vi "Untitled 1.vi"(2 "rate":dbl=2.0, 3 "number of samples":i32=10, 4 "timeout (s)":dbl=10.0 format="%0.2f", 5 "error in":errorcluster, 7 "stop (T)":bool=TRUE) -> (14 "task out":refnum<k21>, 15 "data":dynamicdata(graph), 19 "error out":errorcluster)   [LabVIEW 2024]
doc: "Creates, edits, and runs tasks using NI-DAQmx. Refer to the NI-DAQmx Readme for a complete listing of devices NI-DAQmx supports.\n\nWhen you place this Express VI on the block diagram, the DAQ Assistant launches to create a new task. After you create a task, you can double-click the DAQ Assistant Express VI to edit that task. For continuous measurement or generation, place a while loop around the DAQ Assistant Express VI."
uses:
  <vilib>/DAQmx/read.llb/DAQmx Read.vi
  <vilib>/DAQmx/read.llb/DAQmx Read (Analog 1D Wfm NChan NSamp).vi
  <vilib>/DAQmx/create/channels.llb/DAQmx Create Channel (TEDS-AI-Current-Basic).vi
  <vilib>/DAQmx/create/channels.llb/DAQmx Create Channel (AI-Current-Basic).vi
  <vilib>/DAQmx/create/channels.llb/DAQmx Create Channel (TEDS-AI-Voltage-Basic).vi
  <vilib>/DAQmx/create/channels.llb/DAQmx Create Channel (AI-Voltage-Basic).vi
  <vilib>/DAQmx/configure/timing.llb/DAQmx Timing (Sample Clock).vi
  <vilib>/DAQmx/miscellaneous.llb/DAQmx Fill In Error Info.vi
  <resource>/objmgr/daqmx.rc
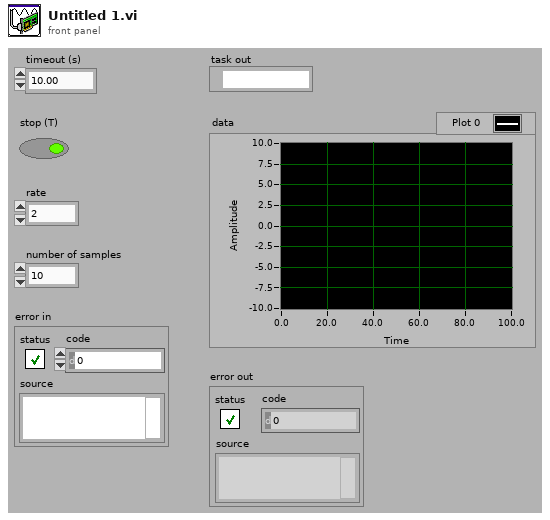
[diagram p1: front panel]
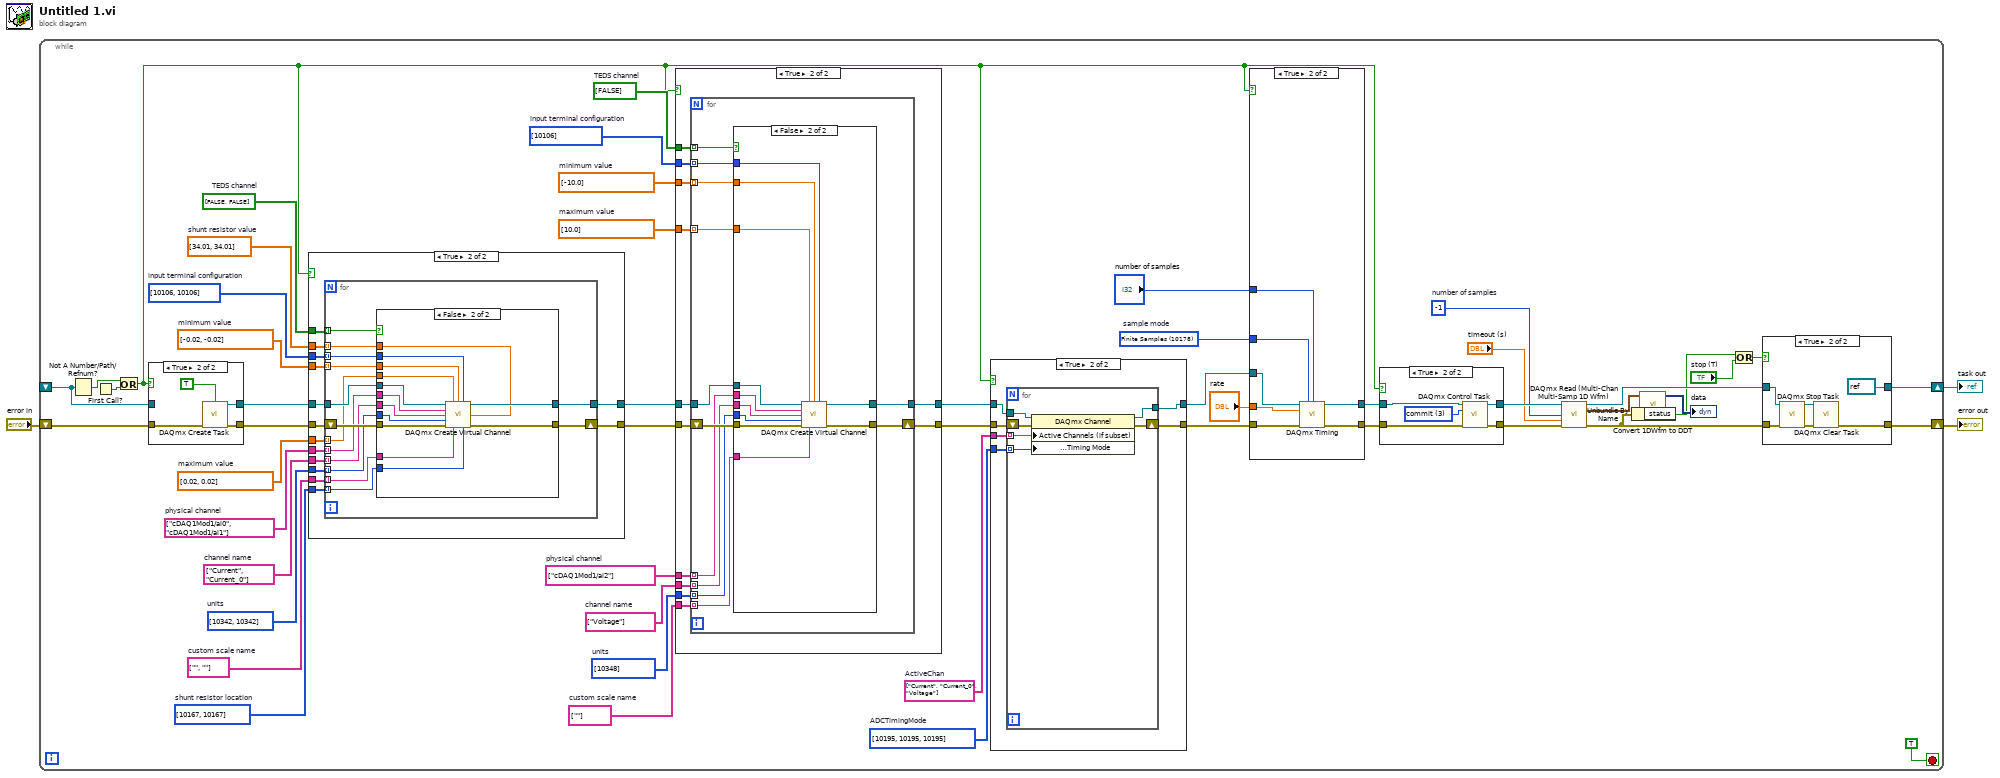
[diagram p0: block diagram]
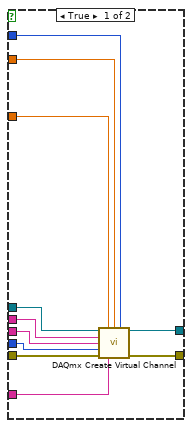
[diagram p7: hidden frame]
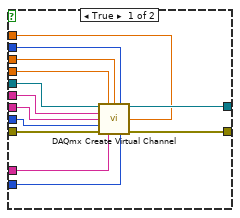
[diagram p9: hidden frame]
diagram:
  n1 = while {
    shift-right: [w10] -> w1
    shift-left: _ -> [w52]
    shift-right: [w8] -> w2
    shift-left: "error in" -> [w53]
    stop <- TRUE stop-if-true
    w14 = -1  # number of samples
    w20 = 10178 items=["Finite Samples"=10178, "Continuous Samples"=10123, "Hardware Timed Single Point"=12522]  # sample mode
    w26 = i32[] [10195, 10195, 10195] items=["High Resolution"=10195, "High Speed"=14712, "Best 50 Hz Rejection"=14713, "Best 60 Hz Rejection"=14714]  # ADCTimingMode
    w27 = string[] ["Current", "Current_0", "Voltage"]  # ActiveChan
    w29 = bool[] [FALSE]  # TEDS channel
    w30 = string[] [""]  # custom scale name
    w31 = i32[] [10348] items=["Volts"=10348, "From TEDS"=12516, "From Custom Scale"=10065]  # units
    w32 = string[] ["Voltage"]  # channel name
    w33 = string[] ["cDAQ1Mod1/ai2"]  # physical channel
    w34 = dbl[] [10.0]  # maximum value
    w35 = dbl[] [-10.0]  # minimum value
    w36 = i32[] [10106] items=["default"=-1, "RSE"=10083, "NRSE"=10078, "Differential"=10106, "Pseudodifferential"=12529]  # input terminal configuration
    w39 = bool[] [FALSE, FALSE]  # TEDS channel
    w41 = i32[] [10167, 10167] items=["Internal"=10200, "External"=10167]  # shunt resistor location
    w40 = dbl[] [34.01, 34.01]  # shunt resistor value
    w42 = string[] ["", ""]  # custom scale name
    w43 = i32[] [10342, 10342] items=["Amps"=10342, "From TEDS"=12516, "From Custom Scale"=10065]  # units
    w44 = string[] ["Current", "Current_0"]  # channel name
    w45 = string[] ["cDAQ1Mod1/ai0", "cDAQ1Mod1/ai1"]  # physical channel
    w46 = dbl[] [0.02, 0.02]  # maximum value
    w47 = dbl[] [-0.02, -0.02]  # minimum value
    w48 = i32[] [10106, 10106] items=["default"=-1, "RSE"=10083, "NRSE"=10078, "Differential"=10106, "Pseudodifferential"=12529]  # input terminal configuration
    n2 = Not A Number/Path/Refnum?(number/path/refnum=w52) -> (NaN/Path/Refnum?=w51:bool)
    n3 = First Call?() -> (First Call?: T/F=w54:bool)
    n4 = Or(x=w51, y=w54) -> (x .or. y?=w19:bool)
    n5 = case shown="True" w19 {
      tunnel: [w199 w203] -> w50
      tunnel: w52 -> [w199 _]
      tunnel: [w198 w202] -> w49
      tunnel: w53 -> [w198 w200]
      frame False {
      }
      frame True {
        n6 = call <vilib>:"DAQmx Create Task.vi"("auto cleanup"=TRUE, "error in"=w200) -> ("task out"=w203:refnum<k21>, "error out"=w202:errorcluster)  [unwired: 12 in]
      }
    }
    n7 = case shown="True" w19 {
      tunnel: [w143 w155] -> w38
      tunnel: w50 -> [w143 w157]
      tunnel: [w142 w154] -> w37
      tunnel: w49 -> [w142 w156]
      tunnel: w48 -> [_ w153]
      tunnel: w47 -> [_ w152]
      tunnel: w46 -> [_ w151]
      tunnel: w45 -> [_ w150]
      tunnel: w44 -> [_ w149]
      tunnel: w43 -> [_ w148]
      tunnel: w42 -> [_ w147]
      tunnel: w41 -> [_ w146]
      tunnel: w40 -> [_ w145]
      tunnel: w39 -> [_ w144]
      frame False {
      }
      frame True {
        n8 = for {
          tunnel: w157 -> [w171]
          tunnel: [w169] -> w155
          tunnel: w153 -> [w167] mode=indexing
          tunnel: w152 -> [w166] mode=indexing
          tunnel: w151 -> [w165] mode=indexing
          tunnel: w150 -> [w164] mode=indexing
          tunnel: w149 -> [w163] mode=indexing
          tunnel: w148 -> [w162] mode=indexing
          tunnel: w147 -> [w161] mode=indexing
          shift-right: [w168] -> w154
          shift-left: w156 -> [w170]
          tunnel: w146 -> [w160] mode=indexing
          tunnel: w145 -> [w159] mode=indexing
          tunnel: w144 -> [w158] mode=indexing
          n9 = case shown="False" w158 {
            tunnel: w171 -> [w184 w197]
            tunnel: w170 -> [w183 w196]
            tunnel: [w182 w195] -> w169
            tunnel: [w181 w194] -> w168
            tunnel: w167 -> [w180 w193]
            tunnel: w166 -> [w179 w192]
            tunnel: w165 -> [w178 w191]
            tunnel: w164 -> [w177 w190]
            tunnel: w163 -> [w176 w189]
            tunnel: w162 -> [w175 w188]
            tunnel: w161 -> [w174 w187]
            tunnel: w160 -> [w173 w186]
            tunnel: w159 -> [w172 w185]
            frame True {
              n10 = call-poly <vilib>:"DAQmx Create Virtual Channel.vi"("task in"=w184, "maximum value"=w178, "minimum value"=w179, "input terminal configuration"=w180, "physical channels"=w177, "name to assign"=w176, "external shunt resistor value"=w172, "units"=w175, "error in"=w183, "custom scale name"=w174, "shunt resistor location"=w173) -> ("task out"=w182:refnum<k21>, "error out"=w181:errorcluster)  [unwired: 3 in]
            }
            frame False {
              n11 = call-poly <vilib>:"DAQmx Create Virtual Channel.vi"("task in"=w197, "maximum value"=w191, "minimum value"=w192, "input terminal configuration"=w193, "physical channels"=w190, "name to assign"=w189, "external shunt resistor value"=w185, "units"=w188, "error in"=w196, "custom scale name"=w187, "shunt resistor location"=w186) -> ("task out"=w195:refnum<k21>, "error out"=w194:errorcluster)  [unwired: 3 in]
            }
          }
        }
      }
    }
    n12 = case shown="True" w19 {
      tunnel: [w95 w105] -> w25
      tunnel: w38 -> [w95 w107]
      tunnel: [w94 w104] -> w28
      tunnel: w37 -> [w94 w106]
      tunnel: w36 -> [_ w103]
      tunnel: w35 -> [_ w102]
      tunnel: w34 -> [_ w101]
      tunnel: w33 -> [_ w100]
      tunnel: w32 -> [_ w99]
      tunnel: w31 -> [_ w98]
      tunnel: w30 -> [_ w97]
      tunnel: w29 -> [_ w96]
      frame False {
      }
      frame True {
        n13 = for {
          tunnel: w107 -> [w119]
          tunnel: [w117] -> w105
          tunnel: w103 -> [w115] mode=indexing
          tunnel: w102 -> [w114] mode=indexing
          tunnel: w101 -> [w113] mode=indexing
          tunnel: w100 -> [w112] mode=indexing
          tunnel: w99 -> [w111] mode=indexing
          tunnel: w98 -> [w110] mode=indexing
          tunnel: w97 -> [w109] mode=indexing
          shift-right: [w116] -> w104
          shift-left: w106 -> [w118]
          tunnel: w96 -> [w108] mode=indexing
          n14 = case shown="False" w108 {
            tunnel: w119 -> [w130 w141]
            tunnel: w118 -> [w129 w140]
            tunnel: [w128 w139] -> w117
            tunnel: [w127 w138] -> w116
            tunnel: w115 -> [w126 w137]
            tunnel: w114 -> [w125 w136]
            tunnel: w113 -> [w124 w135]
            tunnel: w112 -> [w123 w134]
            tunnel: w111 -> [w122 w133]
            tunnel: w110 -> [w121 w132]
            tunnel: w109 -> [w120 w131]
            frame True {
              n15 = call-poly <vilib>:"DAQmx Create Virtual Channel.vi"("task in"=w130, "maximum value"=w124, "minimum value"=w125, "input terminal configuration"=w126, "physical channels"=w123, "name to assign"=w122, "units"=w121, "error in"=w129, "custom scale name"=w120) -> ("task out"=w128:refnum<k21>, "error out"=w127:errorcluster)  [unwired: 5 in]
            }
            frame False {
              n16 = call-poly <vilib>:"DAQmx Create Virtual Channel.vi"("task in"=w141, "maximum value"=w135, "minimum value"=w136, "input terminal configuration"=w137, "physical channels"=w134, "name to assign"=w133, "units"=w132, "error in"=w140, "custom scale name"=w131) -> ("task out"=w139:refnum<k21>, "error out"=w138:errorcluster)  [unwired: 5 in]
            }
          }
        }
      }
    }
    n17 = case shown="True" w19 {
      tunnel: [w81 w84] -> w24
      tunnel: w25 -> [w81 w87]
      tunnel: [w80 w85] -> w23
      tunnel: w28 -> [w80 w86]
      tunnel: w27 -> [_ w83]
      tunnel: w26 -> [_ w82]
      frame False {
      }
      frame True {
        n18 = for {
          tunnel: w87 -> [w93]
          shift-right: [w91] -> w85
          shift-left: w86 -> [w88]
          tunnel: [w92] -> w84
          tunnel: w83 -> [w90] mode=indexing
          tunnel: w82 -> [w89] mode=indexing
          n19 = property class="DAQmx Channel"(reference=w93, error in=w88, "Active Channels (if subset)"=w90, "Analog Input:General Properties:Digitizer/ADC:Timing Mode"=w89) -> (reference out=w92:refnum<k21>, error out=w91:errorcluster)
        }
      }
    }
    n20 = case shown="True" w19 {
      tunnel: [w72 w74] -> w18
      tunnel: w24 -> [w72 w77]
      tunnel: [w71 w73] -> w17
      tunnel: w23 -> [w71 w75]
      tunnel: "number of samples" -> [_ w79]
      tunnel: w20 -> [_ w78]
      tunnel: "rate" -> [_ w76]
      frame False {
      }
      frame True {
        n21 = call-poly <vilib>:"DAQmx Timing.vi"("task/channels in"=w77, "sample mode"=w78, "samples per channel"=w79, "rate"=w76, "error in"=w75) -> ("task out"=w74:refnum<k21>, "error out"=w73:errorcluster)  [unwired: 9 in]
      }
    }
    n22 = case shown="True" w19 {
      tunnel: [w65 w69] -> w16
      tunnel: w18 -> [w65 w70]
      tunnel: [w64 w67] -> w15
      tunnel: w17 -> [w64 w68]
      frame False {
      }
      frame True {
        w66 = 3 items=["verify"=2, "reserve"=4, "commit"=3, "unreserve"=5, "abort"=6] ("action")
        n23 = call <vilib>:"DAQmx Control Task.vi"("task/channels in"=w70, "action"=w66, "error in"=w68) -> ("task out"=w69:refnum<k21>, "error out"=w67:errorcluster)  [unwired: 11 in]
      }
    }
    n24 = call-poly "DAQmx Read (Multi-Chan Multi-Samp 1D Wfm).vi"("task/channels in"=w16, "number of samples per channel"=w14, "timeout"="timeout (s)", "error in"=w15) -> ("task out"=w9:refnum<k21>, "data"=w13:waveform(dbl)[], "error out"=w7:errorcluster)  [unwired: 9 in]
    n25 = Unbundle By Name(w7) -> ("status"=w6:bool)
    n26 = call <vilib>:"Convert 1DWfm to DDT.vi"("Array of Waveforms"=w13) -> ("Dynamic Data Type"=→"data":dynamicdata)  [unwired: 3 in]
    n27 = Or(x=w6, y="stop (T)") -> (x .or. y?=w4:bool)
    n28 = case shown="True" w4 {
      tunnel: [w57 refnum<k21> refnum ("task in")] -> w10
      tunnel: w9 -> [w57 w63]
      tunnel: [w56 w60] -> w8
      tunnel: w7 -> [w56 w62]
      frame False {
      }
      frame True {
        n29 = call <vilib>:"DAQmx Stop Task.vi"("task/channels in"=w63, "error in"=w62) -> ("task out"=w59:refnum<k21>, "error out"=w61:errorcluster)  [unwired: 12 in]
        n30 = call <vilib>:"DAQmx Clear Task.vi"("task in"=w59, "error in"=w61) -> ("error out"=w60:errorcluster)  [unwired: 13 in]
      }
    }
  }
  "error out" <- w2
  "task out" <- w1
